vi "BiaxGlobals (16chan).vi"() -> ()   [LabVIEW 2013]
panel:
  in  "Samp in array 0":i32
  in  "Samp in array":i32
  in  "Accum Time":dbl format="%.2f"
  in  "Rec Rate case":i32
  in  "Var #Samples2Ave":i32
  in  "Var Rec Rate":i32
  in  "Acquisition factor":i32
  in  "#Scans2Average":i16
  out "Counter2":i16
  out "Time to Screen dump":i16
  out "stop":bool
  in  "Rec Rate (samp/s)":i32
  in  "Countdown":i32
  in  "Sample write number":i16
  in  "Time interval to write to disk (s)":i32
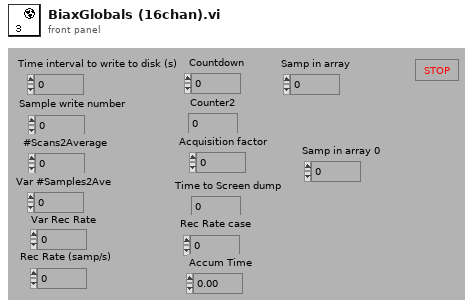
[diagram p1: front panel]
diagram:
